vi "Write Register.vi"(3 "Write Data In":u8, 4 "Write Address":u8 format="%x", 5 "Mouse Sensor In":T1) -> (2 "Mouse Sensor Out":T1)   [LabVIEW 2012, in "Mouse IO.lvlib"]
uses:
  Mouse IO.lvlib
panel:
  # "Mouse Interface\n===\nWrite data to a mouse register"
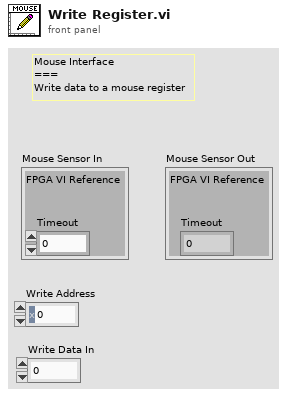
[diagram p1: front panel]
types:
  T1 = cluster{"FPGA VI Reference":refnum<k20>, "Timeout":i32}
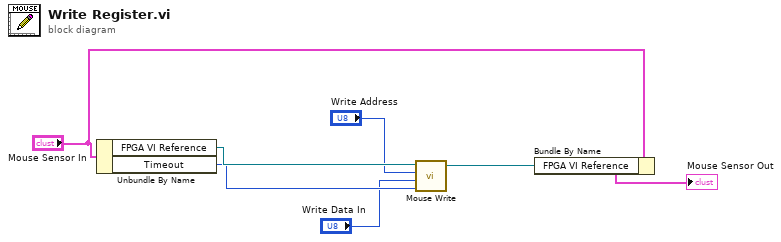
[diagram p0: block diagram]
diagram:
  n1 = Unbundle By Name("Mouse Sensor In") -> ("FPGA VI Reference"=w7:refnum<k20>, "Timeout"=w6:i32)
  n2 = call "Mouse Write.vi"("Timeout (ms)"=w6, "Write Data In"="Write Data In", "Write Address"="Write Address", "FPGA VI Reference In"=w7) -> ("FPGA VI Reference Out"=w3:refnum<k20>)  [unwired: 1 in, 1 out]
  n3 = Bundle By Name(cluster="Mouse Sensor In", "FPGA VI Reference"=w3) -> (→"Mouse Sensor Out":T1)
